vi "Tools_System CPU Usage Init.vi"(8 "error in (no error)":errorcluster) -> (0 "error out":errorcluster, 3 "CPU Usage Ref":T1)   [LabVIEW 2015, in "Performance.lvlib"]
doc: "Initialize the CPU Usage monitor functionality."
uses:
  Performance.lvlib
  tools_system CPU Usage Ref.ctl
  pdh.dll
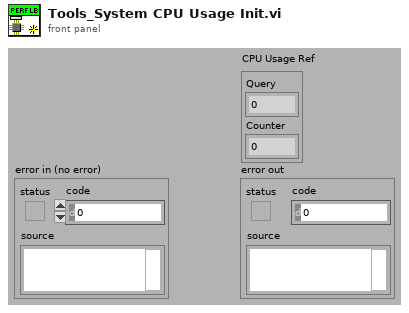
[diagram p1: front panel]
types:
  T1 = typedef "Performance.lvlib/tools_system CPU Usage Ref.ctl" = cluster{"Query":u32, "Counter":u32}
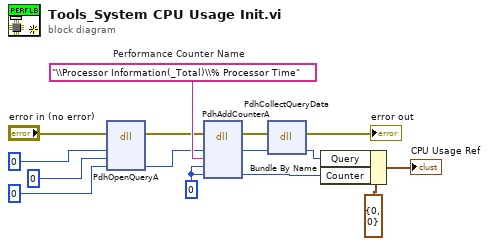
[diagram p0: block diagram]
diagram:
  w15 = "\\Processor Information(_Total)\\% Processor Time"  # Performance Counter Name
  w14 = u32 0 ("phQuery")
  n1 = dll-call lib="pdh.dll" fn="PdhOpenQueryA"(error in="error in (no error)", "szDataSource"=u8 0, "dwUserData"=u32 0, "phQuery"=u32 0) -> (error out=w10:errorcluster, "phQuery"=w9:u32)  [unwired: 5 in, 1 out]
  n2 = dll-call lib="pdh.dll" fn="PdhAddCounterA"(error in=w10, "hQuery"=w9, "szFullCounterPath"=w15, "dwUserData"=w14, "phCounter"=w14) -> (error out=w11:errorcluster, "hQuery"=w12:u32, "phCounter"=w3:u32)  [unwired: 5 in, 1 out]
  n3 = dll-call lib="pdh.dll" fn="PdhCollectQueryData"(error in=w11, "hQuery"=w12) -> (error out=→"error out":errorcluster, "hQuery"=w4:u32)  [unwired: 3 in, 1 out]
  n4 = Bundle By Name(cluster=T1 {"Query"=0, "Counter"=0} ("CPU Usage Ref"), "Query"=w4, "Counter"=w3) -> (→"CPU Usage Ref":T1)
